vi "lithographyTutorial.vi"() -> ()   [LabVIEW 2016]
uses:
  Controls/Tutorial_control.ctl
panel:
  in  "Status":string
  in  "Litho":refnum<k7>
  in  "Application":refnum<k7>
  in  "Scan":refnum<k7>
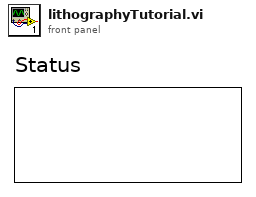
[diagram p1: front panel]
types:
  T1 = typedef "Tutorial_control.ctl" = enum16{"Start", "init_var", "clear_litho", "add_cmds", "set_param", "move_lwr_tip", "draw_square", "retract_tip", "move_center", "start_litho", "End"}
  T2 = cluster{"Application":refnum<k7>, "Scan":refnum<k7>, "Litho":refnum<k7>, "CenterPosY":dbl, "CenterPosX":dbl, "TipSpeed":dbl}
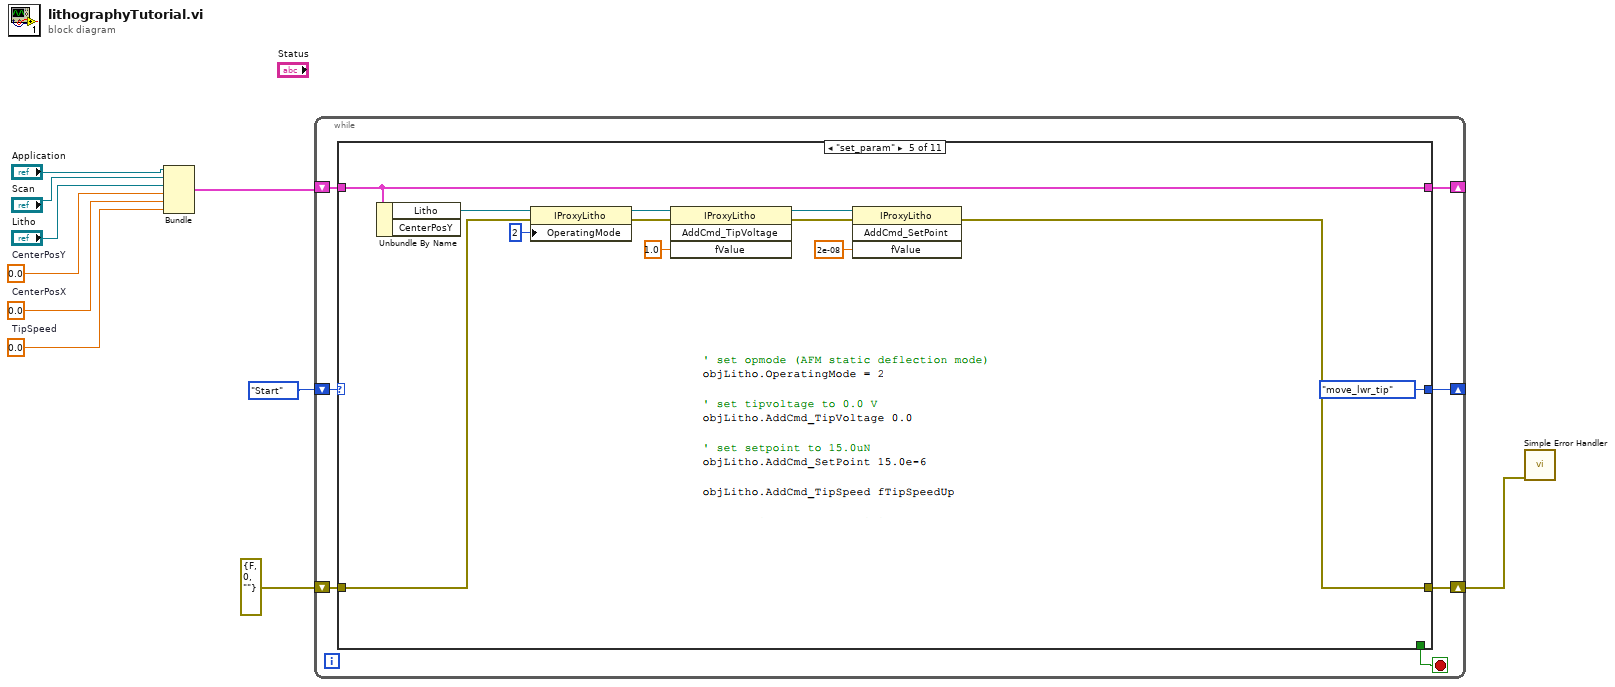
[diagram p0: block diagram]
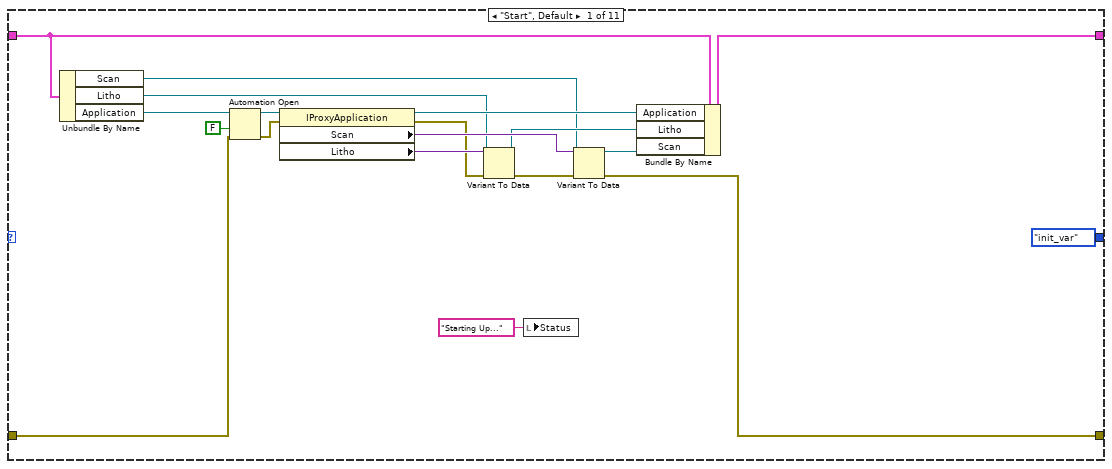
[diagram p2: hidden frame]
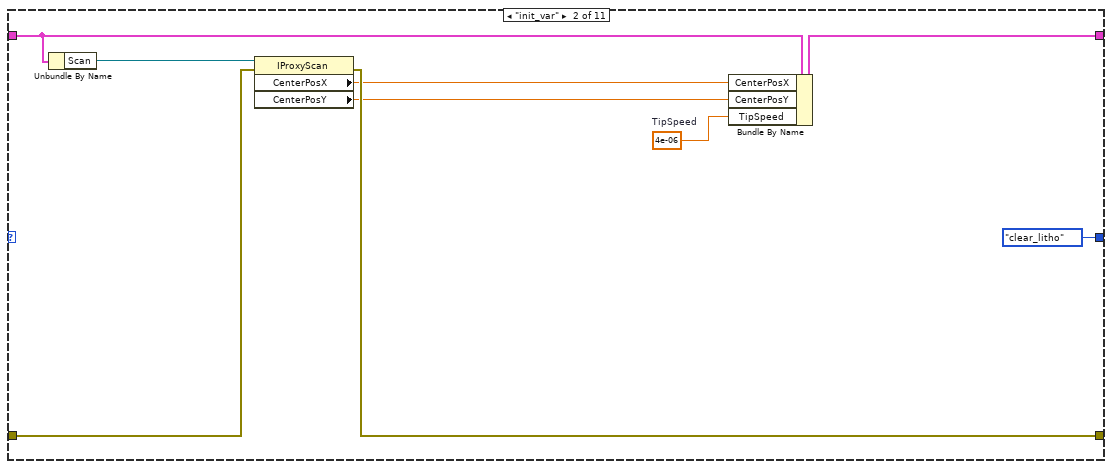
[diagram p3: hidden frame]
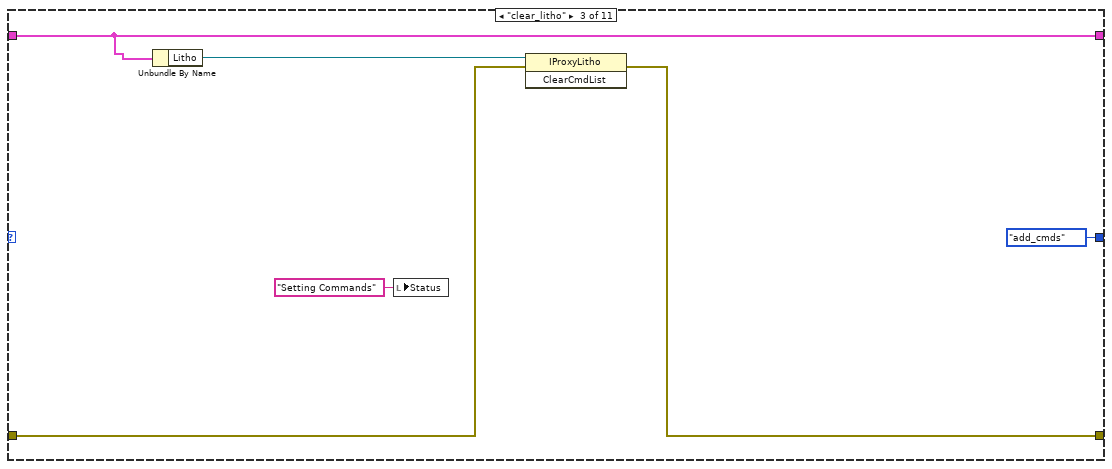
[diagram p4: hidden frame]
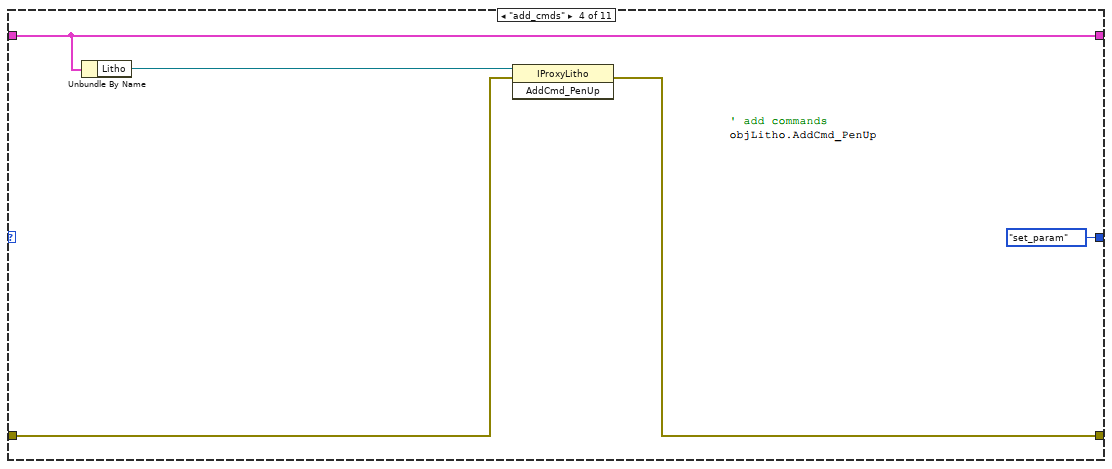
[diagram p5: hidden frame]
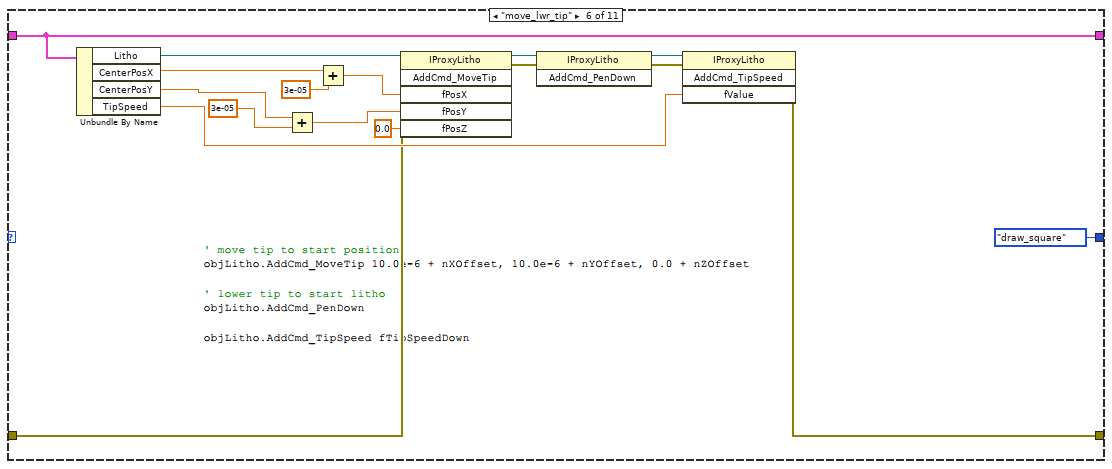
[diagram p6: hidden frame]
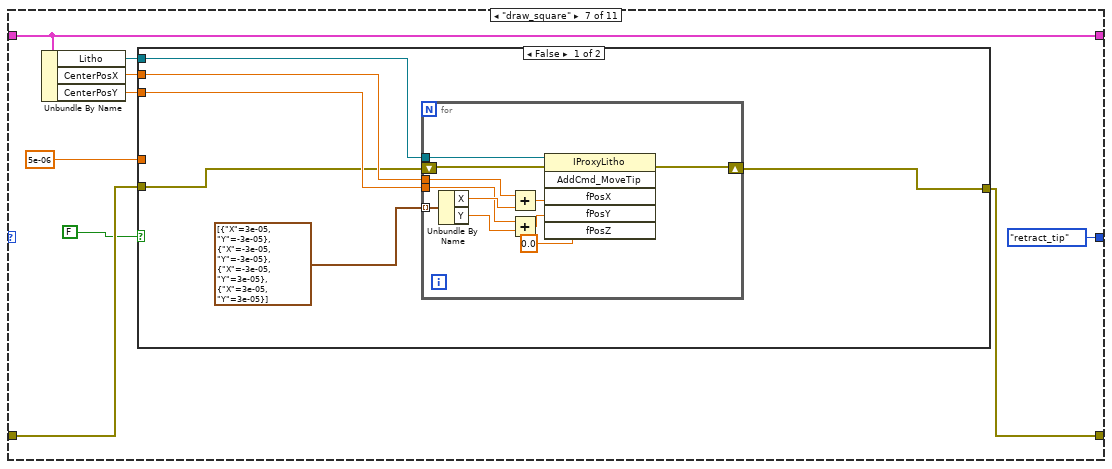
[diagram p7: hidden frame]
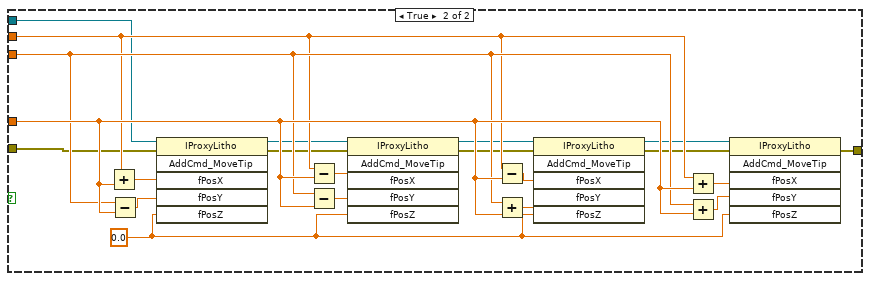
[diagram p8: hidden frame]
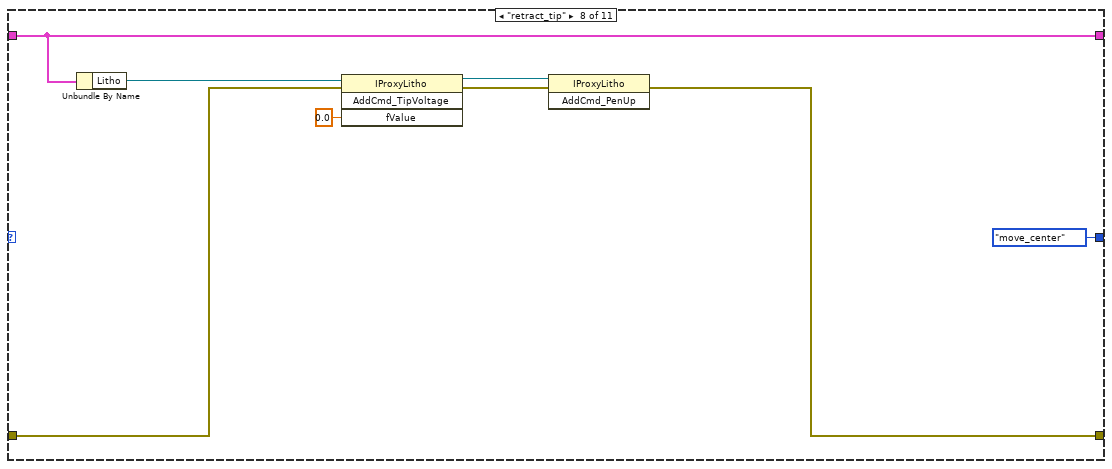
[diagram p9: hidden frame]
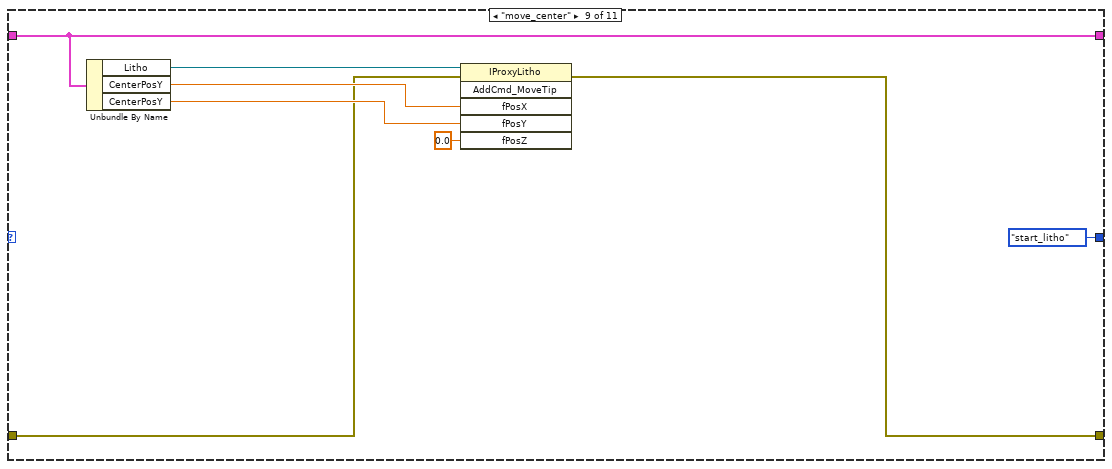
[diagram p10: hidden frame]
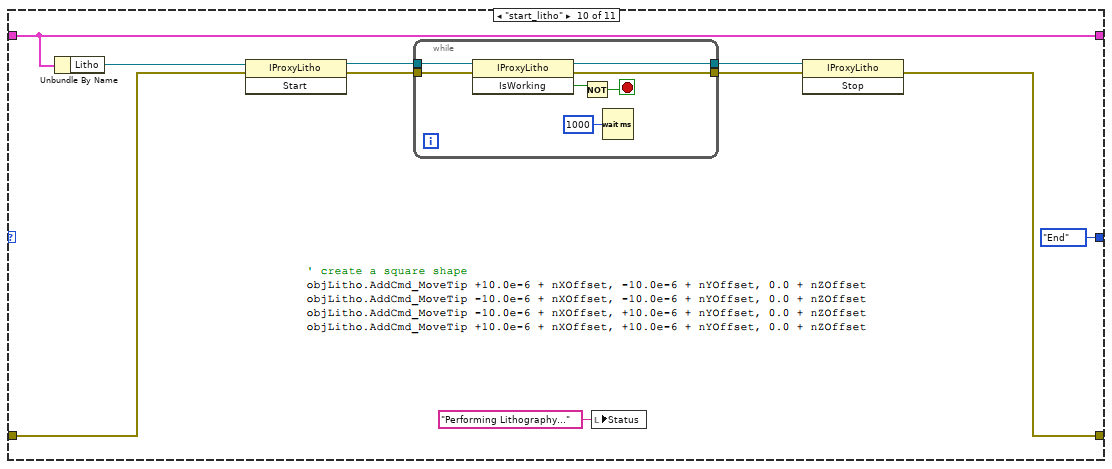
[diagram p11: hidden frame]
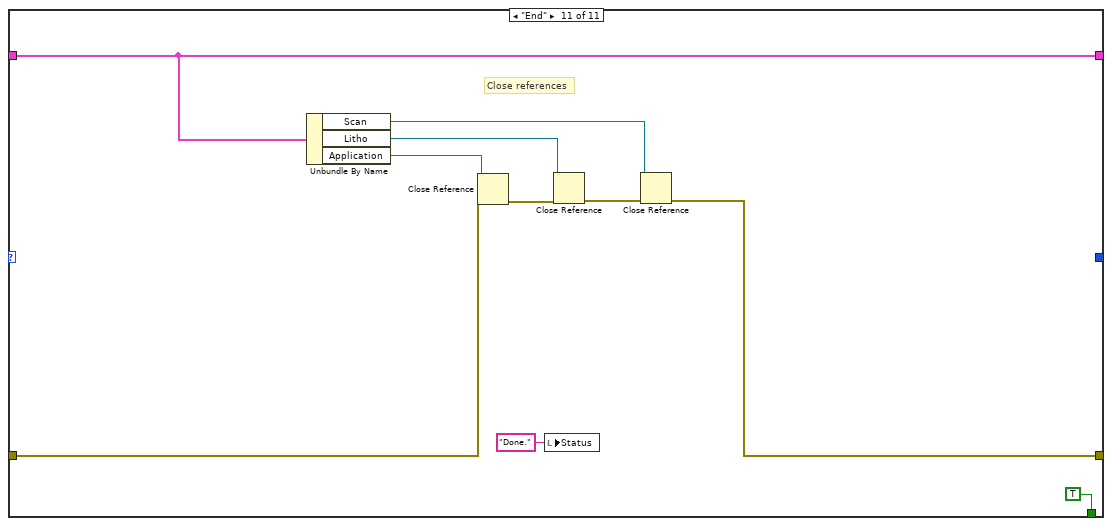
[diagram p12: hidden frame]
diagram:
  w2 = 0.0  # TipSpeed
  w5 = 0.0  # CenterPosY
  w4 = 0.0  # CenterPosX
  n1 = Bundle("Application"="Application", "Scan"="Scan", "Litho"="Litho", "CenterPosY"=w5, "CenterPosX"=w4, "TipSpeed"=w2) -> (w3:T2)  [unwired: 1 in]
  n2 = while {
    shift-right: [w15] -> _
    shift-left: w3 -> [w16]
    shift-right: [w13] -> w1
    shift-left: errorcluster {"status"=FALSE, "code"=0, "source"=""} ("error in (no error)") -> [w14]
    shift-right: [w12] -> _
    shift-left: Tutorial_control."Start" -> [w17]
    stop <- w11 stop-if-true
    n3 = case shown="\"set_param\"" w17 {
      tunnel: w16 -> [w25 w43 w50 w56 w67 w84 w93 w139 w148 w157 w171]
      tunnel: [w24 w42 w50 w56 w67 w84 w93 w139 w148 w157 w171] -> w15
      tunnel: [w19 w40 w47 w53 w57 w69 w91 w138 w142 w149 w167] -> w13
      tunnel: w14 -> [w20 w41 w48 w54 w58 w70 w87 w136 w143 w153 w168]
      tunnel: [Tutorial_control."init_var" Tutorial_control."clear_litho" Tutorial_control."add_cmds" Tutorial_control."set_param" Tutorial_control."move_lwr_tip" Tutorial_control."draw_square" Tutorial_control."retract_tip" Tutorial_control."move_center" Tutorial_control."start_litho" Tutorial_control."End" _] -> w12
      tunnel: [_ _ _ _ _ _ _ _ _ _ TRUE] -> w11
      frame "Start", Default {
        n4 = Unbundle By Name(w25) -> ("Scan"=w29:refnum<k7>, "Litho"=w28:refnum<k7>, "Application"=w26:refnum<k7>)
        n5 = Automation Open(error in (no error)=w20, Automation Refnum=w26, 9:FALSE ("open new instance (false)")) -> (Automation Refnum=w27:refnum<k7>, error out=w21:errorcluster)  [unwired: 1 in]
        n6 = property class="IProxyApplication"(reference=w27, error in=w21) -> (reference out=w30:refnum<k7>, error out=w22:errorcluster, "Scan"=w33:variant, "Litho"=w34:variant)
        n7 = Variant To Data(error in=w22, type=w28, Variant=w34) -> (data=w31:refnum<k7>, error out=w23:errorcluster)
        n8 = local write "Status"("Starting Up..." ("Status")) -> ()
        n9 = Variant To Data(error in=w23, type=w29, Variant=w33) -> (data=w32:refnum<k7>, error out=w19:errorcluster)
        n10 = Bundle By Name(cluster=w25, "Application"=w30, "Litho"=w31, "Scan"=w32) -> (w24:T2)
      }
      frame "init_var" {
        w39 = 4e-06  # TipSpeed
        n11 = Unbundle By Name(w43) -> ("Scan"=w44:refnum<k7>)
        n12 = property class="IProxyScan"(reference=w44, error in=w41) -> (error out=w40:errorcluster, "CenterPosX"=w38:dbl, "CenterPosY"=w37:dbl)  [unwired: 1 out]
        n13 = Bundle By Name(cluster=w43, "CenterPosX"=w38, "CenterPosY"=w37, "TipSpeed"=w39) -> (w42:T2)
      }
      frame "clear_litho" {
        n14 = Unbundle By Name(w50) -> ("Litho"=w49:refnum<k7>)
        n15 = local write "Status"("Setting Commands" ("Status")) -> ()
        n16 = invoke class="IProxyLitho" method="ClearCmdList"(reference=w49, error in=w48) -> (error out=w47:errorcluster)  [unwired: 1 in, 2 out]
      }
      frame "add_cmds" {
        n17 = Unbundle By Name(w56) -> ("Litho"=w55:refnum<k7>)
        n18 = invoke class="IProxyLitho" method="AddCmd_PenUp"(reference=w55, error in=w54) -> (error out=w53:errorcluster)  [unwired: 1 in, 2 out]
      }
      frame "set_param" {
        n19 = Unbundle By Name(w67) -> ("Litho"=w66:refnum<k7>)  [unwired: 1 out]
        n20 = property class="IProxyLitho"(reference=w66, error in=w58, "OperatingMode"=2) -> (reference out=w64:refnum<k7>, error out=w63:errorcluster)
        n21 = invoke class="IProxyLitho" method="AddCmd_TipVoltage"(reference=w64, error in=w63, "fValue"=1.0) -> (reference out=w61:refnum<k7>, error out=w60:errorcluster)  [unwired: 1 in, 2 out]
        n22 = invoke class="IProxyLitho" method="AddCmd_SetPoint"(reference=w61, error in=w60, "fValue"=2e-08) -> (error out=w57:errorcluster)  [unwired: 1 in, 3 out]
      }
      frame "move_lwr_tip" {
        n23 = Unbundle By Name(w84) -> ("Litho"=w83:refnum<k7>, "CenterPosX"=w81:dbl, "CenterPosY"=w78:dbl, "TipSpeed"=w71:dbl)
        n24 = Add(x=w78, y=3e-05 ("CenterPosX")) -> (x+y=w77:dbl)
        n25 = Add(x=w81, y=3e-05 ("CenterPosX")) -> (x+y=w80:dbl)
        n26 = invoke class="IProxyLitho" method="AddCmd_MoveTip"(reference=w83, error in=w70, "fPosX"=w80, "fPosY"=w77, "fPosZ"=0.0) -> (reference out=w75:refnum<k7>, error out=w74:errorcluster)  [unwired: 1 in, 4 out]
        n27 = invoke class="IProxyLitho" method="AddCmd_PenDown"(reference=w75, error in=w74) -> (reference out=w73:refnum<k7>, error out=w72:errorcluster)  [unwired: 1 in, 1 out]
        n28 = invoke class="IProxyLitho" method="AddCmd_TipSpeed"(reference=w73, error in=w72, "fValue"=w71) -> (error out=w69:errorcluster)  [unwired: 1 in, 3 out]
      }
      frame "draw_square" {
        n29 = Unbundle By Name(w93) -> ("Litho"=w88:refnum<k7>, "CenterPosX"=w89:dbl, "CenterPosY"=w90:dbl)
        n30 = case shown="False" FALSE {
          tunnel: 5e-06 ("fPosX") -> [_ w126]
          tunnel: [w95 w122] -> w91
          tunnel: w90 -> [w98 w121]
          tunnel: w89 -> [w99 w120]
          tunnel: w88 -> [w97 w119]
          tunnel: w87 -> [w96 w118]
          frame False {
            n31 = for {
              tunnel: cluster{"X":dbl, "Y":dbl}[] [{"X"=3e-05, "Y"=-3e-05}, {"X"=-3e-05, "Y"=-3e-05}, {"X"=-3e-05, "Y"=3e-05}, {"X"=3e-05, "Y"=3e-05}] -> [w111] mode=indexing
              tunnel: w99 -> [w108]
              tunnel: w98 -> [w107]
              tunnel: w97 -> [w103]
              shift-right: [w101] -> w95
              shift-left: w96 -> [w102]
              n32 = Unbundle By Name(w111) -> ("X"=w110:dbl, "Y"=w109:dbl)
              n33 = Add(x=w108, y=w110) -> (x+y=w105:dbl)
              n34 = Add(x=w107, y=w109) -> (x+y=w106:dbl)
              n35 = invoke class="IProxyLitho" method="AddCmd_MoveTip"(reference=w103, error in=w102, "fPosX"=w105, "fPosY"=w106, "fPosZ"=0.0) -> (error out=w101:errorcluster)  [unwired: 1 in, 5 out]
            }
          }
          frame True {
            w123 = 0.0 ("fPosZ")
            n36 = Add(x=w120, y=w126) -> (x+y=w132:dbl)
            n37 = Subtract(x=w121, y=w126) -> (x-y=w131:dbl)
            n38 = invoke class="IProxyLitho" method="AddCmd_MoveTip"(reference=w119, error in=w118, "fPosX"=w132, "fPosY"=w131, "fPosZ"=w123) -> (reference out=w117:refnum<k7>, error out=w116:errorcluster)  [unwired: 1 in, 4 out]
            n39 = Subtract(x=w120, y=w126) -> (x-y=w130:dbl)
            n40 = Subtract(x=w121, y=w126) -> (x-y=w129:dbl)
            n41 = invoke class="IProxyLitho" method="AddCmd_MoveTip"(reference=w117, error in=w116, "fPosX"=w130, "fPosY"=w129, "fPosZ"=w123) -> (reference out=w114:refnum<k7>, error out=w115:errorcluster)  [unwired: 1 in, 4 out]
            n42 = Subtract(x=w120, y=w126) -> (x-y=w128:dbl)
            n43 = Add(x=w121, y=w126) -> (x+y=w127:dbl)
            n44 = invoke class="IProxyLitho" method="AddCmd_MoveTip"(reference=w114, error in=w115, "fPosX"=w128, "fPosY"=w127, "fPosZ"=w123) -> (reference out=w113:refnum<k7>, error out=w112:errorcluster)  [unwired: 1 in, 4 out]
            n45 = Add(x=w120, y=w126) -> (x+y=w125:dbl)
            n46 = Add(x=w121, y=w126) -> (x+y=w124:dbl)
            n47 = invoke class="IProxyLitho" method="AddCmd_MoveTip"(reference=w113, error in=w112, "fPosX"=w125, "fPosY"=w124, "fPosZ"=w123) -> (error out=w122:errorcluster)  [unwired: 1 in, 5 out]
          }
        }
      }
      frame "retract_tip" {
        n48 = Unbundle By Name(w139) -> ("Litho"=w137:refnum<k7>)
        n49 = invoke class="IProxyLitho" method="AddCmd_TipVoltage"(reference=w137, error in=w136, "fValue"=0.0) -> (reference out=w134:refnum<k7>, error out=w135:errorcluster)  [unwired: 1 in, 2 out]
        n50 = invoke class="IProxyLitho" method="AddCmd_PenUp"(reference=w134, error in=w135) -> (error out=w138:errorcluster)  [unwired: 1 in, 2 out]
      }
      frame "move_center" {
        n51 = Unbundle By Name(w148) -> ("Litho"=w147:refnum<k7>, "CenterPosY"=w146:dbl, "CenterPosY"=w145:dbl)
        n52 = invoke class="IProxyLitho" method="AddCmd_MoveTip"(reference=w147, error in=w143, "fPosX"=w146, "fPosY"=w145, "fPosZ"=0.0) -> (error out=w142:errorcluster)  [unwired: 1 in, 5 out]
      }
      frame "start_litho" {
        n53 = Unbundle By Name(w157) -> ("Litho"=w156:refnum<k7>)
        n54 = invoke class="IProxyLitho" method="Start"(reference=w156, error in=w153) -> (reference out=w154:refnum<k7>, error out=w155:errorcluster)  [unwired: 1 in, 1 out]
        n55 = while {
          tunnel: w155 -> [w165]
          tunnel: w154 -> [w164]
          tunnel: [w161] -> w150
          tunnel: [w159] -> w151
          stop <- w162 stop-if-true
          n56 = invoke class="IProxyLitho" method="IsWorking"(reference=w164, error in=w165) -> (reference out=w159:refnum<k7>, error out=w161:errorcluster, "IsWorking"=w163:bool)  [unwired: 1 in]
          n57 = Not(x=w163) -> (.not. x?=w162:bool)
          n58 = Wait (ms)(milliseconds to wait=u32 1000) -> ()  [unwired: 1 out]
        }
        n59 = local write "Status"("Performing Lithography..." ("Status")) -> ()
        n60 = invoke class="IProxyLitho" method="Stop"(reference=w151, error in=w150) -> (error out=w149:errorcluster)  [unwired: 1 in, 2 out]
      }
      frame "End" {
        # "Close references"
        n61 = Unbundle By Name(w171) -> ("Scan"=w172:refnum<k7>, "Litho"=w173:refnum<k7>, "Application"=w174:refnum<k7>)
        n62 = Close Reference(reference=w174, error in (no error)=w168) -> (error out=w169:errorcluster)
        n63 = local write "Status"("Done." ("Status")) -> ()
        n64 = Close Reference(reference=w173, error in (no error)=w169) -> (error out=w170:errorcluster)
        n65 = Close Reference(reference=w172, error in (no error)=w170) -> (error out=w167:errorcluster)
      }
    }
  }
  n66 = call <vilib>:"Simple Error Handler.vi"("error in (no error)"=w1) -> ()  [unwired: 4 in, 5 out]
